vi "GLdrv_Open.vi"   [LabVIEW 2017, in "GL860_Driver.lvlib"]
uses:
  GL860_Driver.lvlib
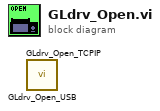
[diagram p0: block diagram]
diagram:
  n1 = call "GLdrv_Open_USB.vi"() -> ()  [unwired: 14 in, 2 out]
  n2 = call "GLdrv_Open_TCPIP.vi"() -> ()  [unwired: 14 in, 2 out]
